vi "StopMotor.vi"(8 "Error In":errorcluster, 11 "Thorlabs In":refnum<class "Thorlabs.lvclass">) -> (0 "Error Out":errorcluster, 3 "Thorlabs Out":refnum<class "Thorlabs.lvclass">)   [LabVIEW 2018, in "Thorlabs.lvlib" / "Thorlabs.lvclass"]
doc: "This VI stops the Motor on the Device immedatiely. \n\nCreator: Slade Jeppesen\nCreated Date: 09/29/20"
uses:
  Thorlabs.lvclass
  Thorlabs.lvclass/Thorlabs.ctl
  3876280e-00b6-43b8-a5f1-c8e8eab95e3f.vi
  C:/AME Test Engineering/LabVIEW/PPLs/Axis/DLLs/ThorLabs.MotionControl.KCube.DCServoCLI.dll
  PPLs/Axis/DLLs/ThorLabs.MotionControl.KCube.DCServoCLI.dll
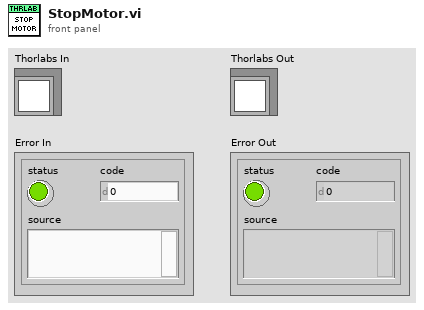
[diagram p1: front panel]
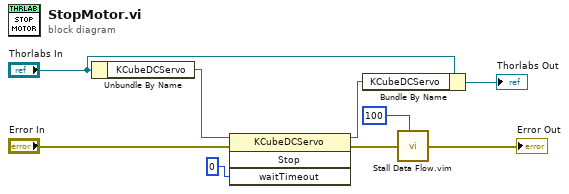
[diagram p0: block diagram]
diagram:
  n1 = Unbundle By Name("Thorlabs In") -> ("KCubeDCServo"=w9:refnum<k24>)
  n2 = invoke class="KCubeDCServo" method="Stop"(reference=w9, error in="Error In", "waitTimeout"=0) -> (reference out=w1:refnum<k24>, error out=w2:errorcluster)  [unwired: 1 in, 2 out]
  n3 = Bundle By Name(cluster="Thorlabs In", "KCubeDCServo"=w1) -> (→"Thorlabs Out":refnum<class "Thorlabs.lvclass">)
  n4 = call "Stall Data Flow.vim"("value in"=w2, "milliseconds to wait"=100 ("waitTimeout")) -> ("value out"=→"Error Out":errorcluster)  [unwired: 1 out]
